vi "variant2Attributes.vi"(0 "HGF_SVDataConverter":refnum<class "HGF_SVDataConverter.lvclass">, 2 "rawData":variant, 3 "typeDescriptor":string, 5 "error in (no error)":errorcluster) -> (14 "HGF_SVDataConverter":refnum<class "HGF_SVDataConverter.lvclass">, 15 "no link":bool, 16 "Parameter":variant, 17 "typeDescriptor":string, 19 "error out":errorcluster)   [LabVIEW 2012, in "HGF_SV.lvlib" / "HGF_SVDataConverter.lvclass"]
doc: "Convert raw data value of variant to variant attributes Pn, n=0,1,2,..."
uses:
  HGF_SVDataConverter.lvclass
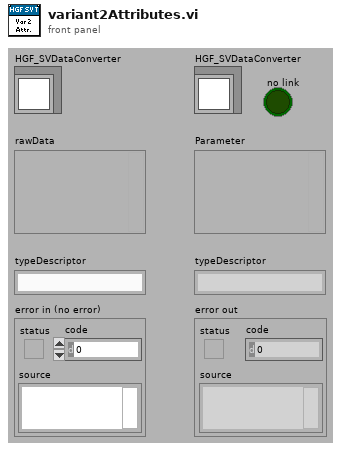
[diagram p1: front panel]
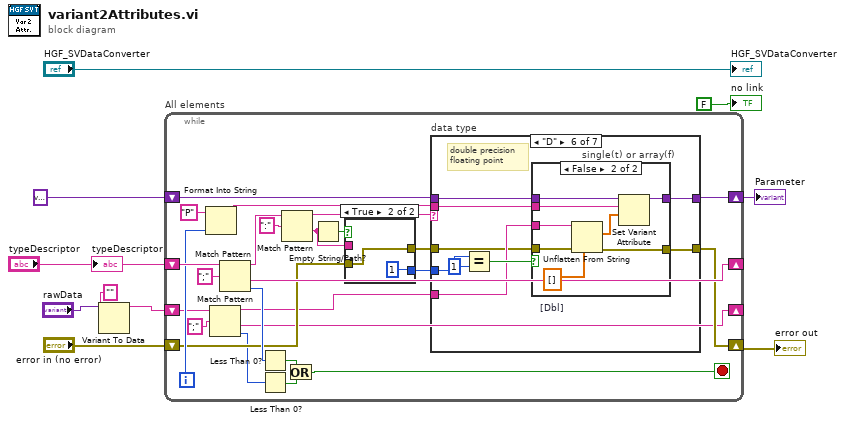
[diagram p0: block diagram]
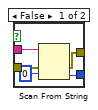
[diagram p2: hidden frame]
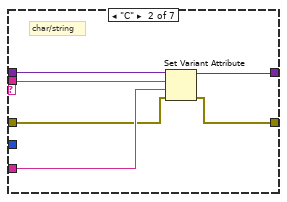
[diagram p4: hidden frame]
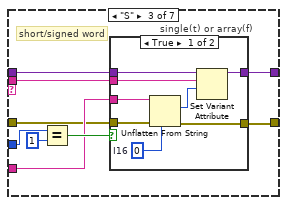
[diagram p5: hidden frame]
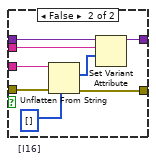
[diagram p6: hidden frame]
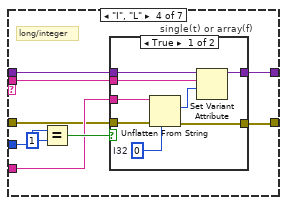
[diagram p7: hidden frame]
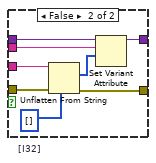
[diagram p8: hidden frame]
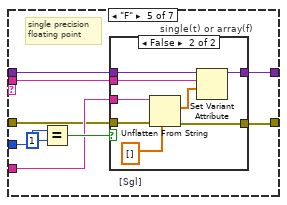
[diagram p9: hidden frame]
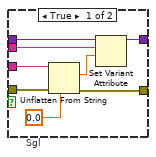
[diagram p10: hidden frame]
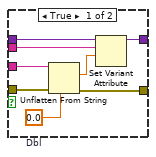
[diagram p11: hidden frame]
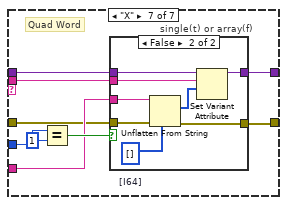
[diagram p12: hidden frame]
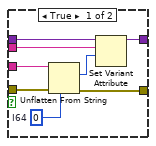
[diagram p13: hidden frame]
diagram:
  n1 = Variant To Data(type="" ("typeDescriptor 2"), Variant="rawData") -> (data=w4:string)  [unwired: 1 in, 1 out]
  n2 = while "All elements" {
    shift-right: [w34] -> _
    shift-left: "typeDescriptor" -> [w36]
    shift-right: [w24] -> w1
    shift-left: variant ("Parameter") -> [w25]
    shift-right: [w21] -> w2
    shift-left: "error in (no error)" -> [w23]
    shift-right: [w17] -> _
    shift-left: w4 -> [w19]
    i -> [w31]
    stop <- w13 stop-if-true
    n3 = Format Into String(initial string="P", w31) -> (resulting string=w26:string)  [unwired: 2 in, 1 out]
    n4 = Match Pattern(string=w19, regular expression=";") -> (before substring=w18:string, after substring=w17:string, offset past match=w16:i32)  [unwired: 2 out]
    n5 = Match Pattern(string=w36, regular expression=";") -> (before substring=w29:string, after substring=w34:string, offset past match=w33:i32)  [unwired: 2 out]
    n6 = Less Than 0?(x=w33) -> (x < 0?=w15:bool)
    n7 = Less Than 0?(x=w16) -> (x < 0?=w14:bool)
    n8 = Match Pattern(string=w29, regular expression=":") -> (before substring=w28:string, after substring=w12:string)  [unwired: 3 out]
    n9 = Or(x=w15, y=w14) -> (x .or. y?=w13:bool)
    n10 = Empty String/Path?(string/path=w12) -> (empty?=w11:bool)
    n11 = case shown="True" w11 {
      tunnel: w12 -> [w41 _]
      tunnel: [w39 1 ("default value 1")] -> w27
      tunnel: w23 -> [w38 w43]
      tunnel: [w37 w43] -> w22
      frame False {
        n12 = Scan From String(input string=w41, error in=w38, default 1=0 ("default value 1")) -> (error out=w37:errorcluster, output 1=w39:i32)  [unwired: 2 in, 2 out]
      }
      frame True {
      }
    }
    n13 = case "data type" shown="\"D\"" w28 {
      tunnel: w18 -> [_ w48 w54 w79 w104 w129 w154]
      tunnel: w27 -> [_ _ w60 w85 w110 w135 w160]
      tunnel: w26 -> [_ w49 w55 w80 w105 w130 w155]
      tunnel: w25 -> [w45 w51 w57 w82 w107 w132 w157]
      tunnel: [w45 w50 w56 w81 w106 w131 w156] -> w24
      tunnel: w22 -> [w44 w47 w53 w78 w103 w128 w153]
      tunnel: [w44 w46 w52 w77 w102 w127 w152] -> w21
      frame Default {
      }
      frame "C" {
        # "char/string"
        n14 = Set Variant Attribute(Variant=w51, name=w49, value=w48, error in=w47) -> (Variant out=w50:variant, error out=w46:errorcluster)  [unwired: 1 out]
      }
      frame "S" {
        # "short/signed word"
        n15 = Equal?(x=w60, y=1) -> (x = y?=w58:bool)
        n16 = case "single(t) or array(f)" shown="True" w58 {
          tunnel: w57 -> [w68 w76]
          tunnel: [w67 w75] -> w56
          tunnel: w55 -> [w66 w74]
          tunnel: w54 -> [w65 w73]
          tunnel: w53 -> [w62 w71]
          tunnel: [w61 w70] -> w52
          frame True {
            w64 = i16 0  # I16
            n17 = Unflatten From String(type=w64, binary string=w65, error in (no error)=w62) -> (value=w63:i16, error out=w61:errorcluster)  [unwired: 3 out]
            n18 = Set Variant Attribute(Variant=w68, name=w66, value=w63) -> (Variant out=w67:variant)  [unwired: 1 in, 2 out]
          }
          frame False {
            w69 = i16[] []  # [I16]
            n19 = Unflatten From String(type=w69, binary string=w73, error in (no error)=w71) -> (value=w72:i16[], error out=w70:errorcluster)  [unwired: 3 out]
            n20 = Set Variant Attribute(Variant=w76, name=w74, value=w72) -> (Variant out=w75:variant)  [unwired: 1 in, 2 out]
          }
        }
      }
      frame "I", "L" {
        # "long/integer"
        n21 = Equal?(x=w85, y=1) -> (x = y?=w83:bool)
        n22 = case "single(t) or array(f)" shown="True" w83 {
          tunnel: w82 -> [w93 w101]
          tunnel: [w92 w100] -> w81
          tunnel: w80 -> [w91 w99]
          tunnel: w79 -> [w90 w98]
          tunnel: w78 -> [w87 w96]
          tunnel: [w86 w95] -> w77
          frame True {
            w89 = 0  # I32
            n23 = Unflatten From String(type=w89, binary string=w90, error in (no error)=w87) -> (value=w88:i32, error out=w86:errorcluster)  [unwired: 3 out]
            n24 = Set Variant Attribute(Variant=w93, name=w91, value=w88) -> (Variant out=w92:variant)  [unwired: 1 in, 2 out]
          }
          frame False {
            w94 = i32[] []  # [I32]
            n25 = Unflatten From String(type=w94, binary string=w98, error in (no error)=w96) -> (value=w97:i32[], error out=w95:errorcluster)  [unwired: 3 out]
            n26 = Set Variant Attribute(Variant=w101, name=w99, value=w97) -> (Variant out=w100:variant)  [unwired: 1 in, 2 out]
          }
        }
      }
      frame "F" {
        # "single precision\nfloating point"
        n27 = Equal?(x=w110, y=1) -> (x = y?=w108:bool)
        n28 = case "single(t) or array(f)" shown="False" w108 {
          tunnel: w107 -> [w118 w126]
          tunnel: [w117 w125] -> w106
          tunnel: w105 -> [w116 w124]
          tunnel: w104 -> [w115 w123]
          tunnel: w103 -> [w112 w121]
          tunnel: [w111 w120] -> w102
          frame True {
            w114 = sgl 0.0  # Sgl
            n29 = Unflatten From String(type=w114, binary string=w115, error in (no error)=w112) -> (value=w113:sgl, error out=w111:errorcluster)  [unwired: 3 out]
            n30 = Set Variant Attribute(Variant=w118, name=w116, value=w113) -> (Variant out=w117:variant)  [unwired: 1 in, 2 out]
          }
          frame False {
            w119 = sgl[] []  # [Sgl]
            n31 = Unflatten From String(type=w119, binary string=w123, error in (no error)=w121) -> (value=w122:sgl[], error out=w120:errorcluster)  [unwired: 3 out]
            n32 = Set Variant Attribute(Variant=w126, name=w124, value=w122) -> (Variant out=w125:variant)  [unwired: 1 in, 2 out]
          }
        }
      }
      frame "D" {
        # "double precision\nfloating point"
        n33 = Equal?(x=w135, y=1) -> (x = y?=w133:bool)
        n34 = case "single(t) or array(f)" shown="False" w133 {
          tunnel: w132 -> [w143 w151]
          tunnel: [w142 w150] -> w131
          tunnel: w130 -> [w141 w149]
          tunnel: w129 -> [w140 w148]
          tunnel: w128 -> [w137 w146]
          tunnel: [w136 w145] -> w127
          frame True {
            w139 = 0.0  # Dbl
            n35 = Unflatten From String(type=w139, binary string=w140, error in (no error)=w137) -> (value=w138:dbl, error out=w136:errorcluster)  [unwired: 3 out]
            n36 = Set Variant Attribute(Variant=w143, name=w141, value=w138) -> (Variant out=w142:variant)  [unwired: 1 in, 2 out]
          }
          frame False {
            w144 = dbl[] []  # [Dbl]
            n37 = Unflatten From String(type=w144, binary string=w148, error in (no error)=w146) -> (value=w147:dbl[], error out=w145:errorcluster)  [unwired: 3 out]
            n38 = Set Variant Attribute(Variant=w151, name=w149, value=w147) -> (Variant out=w150:variant)  [unwired: 1 in, 2 out]
          }
        }
      }
      frame "X" {
        # "Quad Word"
        n39 = Equal?(x=w160, y=1) -> (x = y?=w158:bool)
        n40 = case "single(t) or array(f)" shown="False" w158 {
          tunnel: w157 -> [w168 w176]
          tunnel: [w167 w175] -> w156
          tunnel: w155 -> [w166 w174]
          tunnel: w154 -> [w165 w173]
          tunnel: w153 -> [w162 w171]
          tunnel: [w161 w170] -> w152
          frame True {
            w164 = i64 0  # I64
            n41 = Unflatten From String(type=w164, binary string=w165, error in (no error)=w162) -> (value=w163:i64, error out=w161:errorcluster)  [unwired: 3 out]
            n42 = Set Variant Attribute(Variant=w168, name=w166, value=w163) -> (Variant out=w167:variant)  [unwired: 1 in, 2 out]
          }
          frame False {
            w169 = i64[] []  # [I64]
            n43 = Unflatten From String(type=w169, binary string=w173, error in (no error)=w171) -> (value=w172:i64[], error out=w170:errorcluster)  [unwired: 3 out]
            n44 = Set Variant Attribute(Variant=w176, name=w174, value=w172) -> (Variant out=w175:variant)  [unwired: 1 in, 2 out]
          }
        }
      }
    }
  }
  "error out" <- w2
  "Parameter" <- w1
  "HGF_SVDataConverter" <- "HGF_SVDataConverter"
  "typeDescriptor" <- "typeDescriptor"
  "no link" <- FALSE ("no link")
